vi "Get Operation Mode.vi"(0 "VISA resource name":refnum<visa-resource-name>, 11 "error in (no error)":errorcluster) -> (4 "VISA resource name out":refnum<visa-resource-name>, 6 "Operation Mode":enum16{"Program", "Manual"}(ring), 15 "error out":errorcluster)   [LabVIEW 2020, in "eec 6700.lvlib"]
doc: "Gets the Operation mode (Program, Manual) configured to the Power source instrument."
uses:
  <instrlib>/eec 6700/eec 6700.lvlib
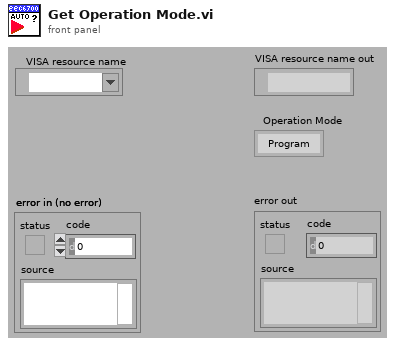
[diagram p1: front panel]
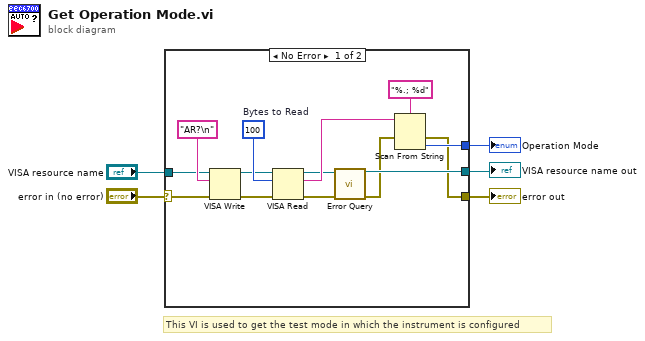
[diagram p0: block diagram]
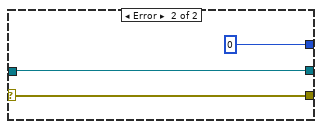
[diagram p2: hidden frame]
diagram:
  # "This VI is used to get the test mode in which the instrument is configured"
  n1 = case shown="No Error" "error in (no error)" {
    selector: "error in (no error)" -> [w18 w22]
    tunnel: [w8 w22] -> w4
    tunnel: [w10 w21] -> w2
    tunnel: "VISA resource name" -> [w17 w21]
    tunnel: [w15 0] -> w1
    frame No Error {
      w14 = u32 100  # Bytes to Read
      n2 = VISA Write(VISA resource name=w17, write buffer="AR?\n", error in (no error)=w18) -> (VISA resource name out=w13:refnum<visa-resource-name>, error out=w12:errorcluster)  [unwired: 1 out]
      n3 = VISA Read(VISA resource name=w13, byte count=w14, error in (no error)=w12) -> (VISA resource name out=w9:refnum<visa-resource-name>, read buffer=w11:string, error out=w7:errorcluster)  [unwired: 1 out]
      n4 = call <instrlib>:"Error Query.vi"("VISA resource name"=w9, "error in (no error)"=w7) -> ("VISA resource name out"=w10:refnum<visa-resource-name>, "error out"=w6:errorcluster)  [unwired: 10 in, 2 out]
      n5 = Scan From String(format string="%.; %d", input string=w11, error in=w6) -> (error out=w8:errorcluster, output 1=w15:i32)  [unwired: 2 in, 2 out]
    }
    frame Error {
    }
  }
  "error out" <- w4
  "VISA resource name out" <- w2
  "Operation Mode" <- w1
